vi "Test Missing VIs.vi"(8 "error in":errorcluster, 11 "My Computer":refnum<vi>) -> (0 "error out":errorcluster, 4 "Missing items":path[](array[path]), 5 "Pass":bool)   [LabVIEW 2020, in "Missing in Project Tests.lvlib"]
doc: "Tests to make sure all VIs and Ctls defined in the project are saved to disk."
uses:
  Missing in Project Tests.lvlib
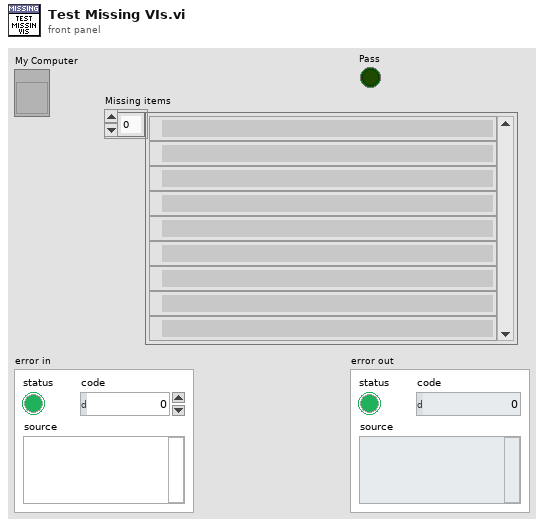
[diagram p1: front panel]
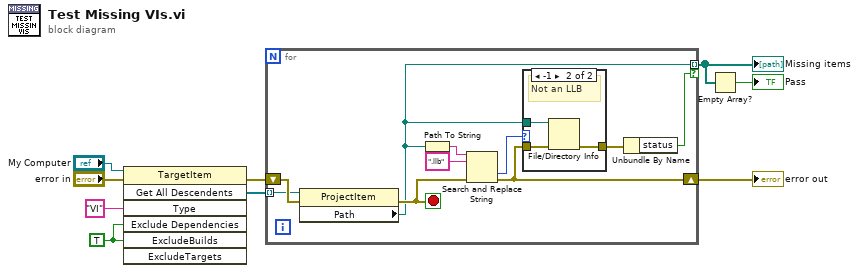
[diagram p0: block diagram]
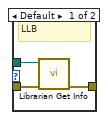
[diagram p2: hidden frame]
diagram:
  w2 = TRUE ("ExcludeBuilds")
  n1 = invoke on="Invoke Node" class="TargetItem" method="Get All Descendents"(reference="My Computer", error in="error in", "Type"="VI", "Exclude Dependencies"=w2, "ExcludeBuilds"=w2) -> (error out=w9:errorcluster, "All Descendents"=w5:refnum<vi>[])  [unwired: 2 in, 5 out]
  n2 = for {
    tunnel: w5 -> [w15] mode=indexing
    shift-right: [w16] -> w8
    shift-left: w9 -> [w18]
    tunnel: [w10] -> w4 mode=indexing if=w14
    stop <- w17 stop-if-true
    n3 = property on="Property Node" class="ProjectItem"(reference=w15, error in=w18) -> (error out=w17:errorcluster, "Path"=w10:path)  [unwired: 1 out]
    n4 = Path To String(path=w10) -> (string=w13:string)
    n5 = Search and Replace String(input string=w13, search string=".llb", error in=w17) -> (offset past replacement=w11:i32, error out=w16:errorcluster)  [unwired: 5 in, 2 out]
    n6 = case shown="-1" w11 {
      tunnel: w16 -> [w22 w25]
      tunnel: [w21 w24] -> w19
      tunnel: w10 -> [w20 w23]
      frame Default {
        # "LLB"
        n7 = call <vilib>:"Librarian Get Info.vi"("error in (no error)"=w22, "path"=w20) -> ("error out"=w21:errorcluster)  [unwired: 7 in, 2 out]
      }
      frame -1 {
        # "Not an LLB"
        n8 = File/Directory Info(path=w23, error in=w25) -> (error out=w24:errorcluster)  [unwired: 6 out]
      }
    }
    n9 = Unbundle By Name(w19) -> ("status"=w14:bool)
  }
  "Missing items" <- w4
  "error out" <- w8
  n10 = Empty Array?(array=w4) -> (empty?=→"Pass":bool)
